vi "everest_loop_test.vi"(1 "error in (no error)":errorcluster, 2 "VISA resource name":refnum<visa-resource-name>="COM3") -> (0 "error out":errorcluster caption="错误输出")   [LabVIEW 2015]
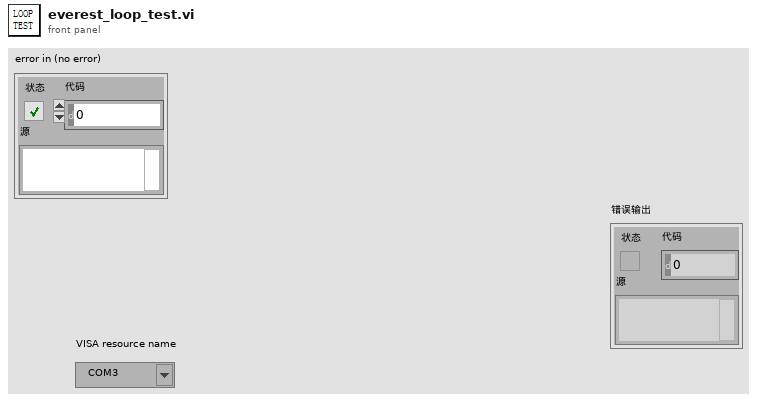
[diagram p1: front panel]
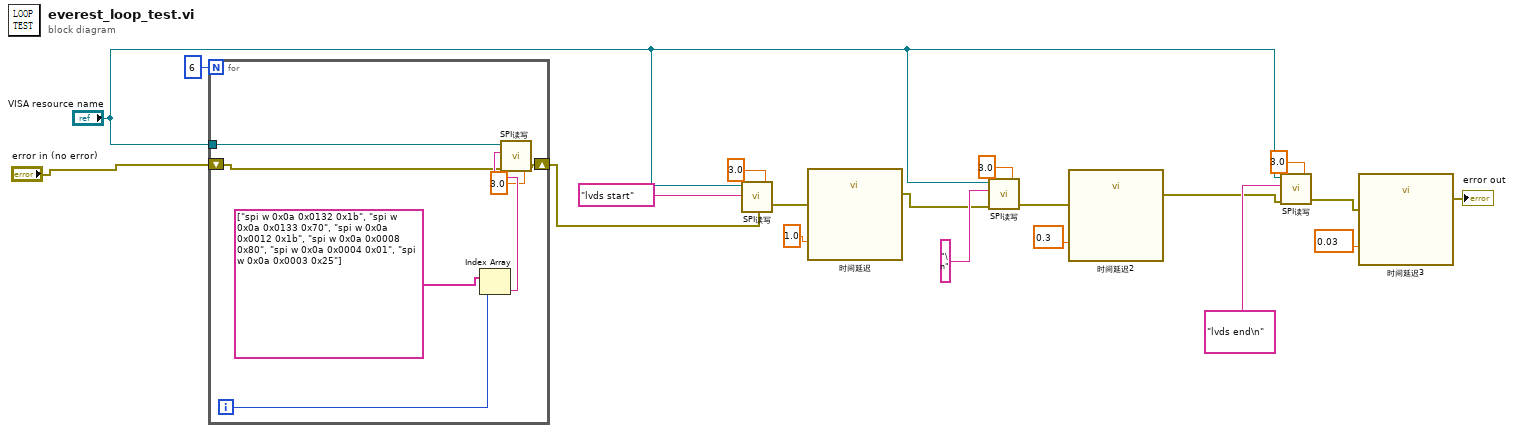
[diagram p0: block diagram]
diagram:
  n1 = for {
    N: 6 -> [_]
    tunnel: "VISA resource name" -> [w23]
    shift-right: [w21] -> w17
    shift-left: "error in (no error)" -> [w22]
    i -> [w25]
    n2 = Index Array(array=string[] ["spi w 0x0a 0x0132 0x1b", "spi w 0x0a 0x0133 0x70", "spi w 0x0a 0x0012 0x1b", "spi w 0x0a 0x0008 0x80", "spi w 0x0a 0x0004 0x01", "spi w 0x0a 0x0003 0x25"], index=w25) -> (element=w24:string)
    n3 = call "SPI读写.vi"("DELAY"=3.0, "error in (no error)"=w22, "往芯片写数据"=w24, "VISA resource name"=w23) -> ("error out"=w21:errorcluster)  [unwired: 1 in, 1 out]
  }
  n4 = call "SPI读写.vi"("DELAY"=3.0, "error in (no error)"=w17, "往芯片写数据"="lvds start", "VISA resource name"="VISA resource name") -> ("error out"=w16:errorcluster)  [unwired: 1 in, 1 out]
  n5 = call "时间延迟"("error in (no error)"=w16, "Delay Time (s)"=1.0) -> ("error out"=w13:errorcluster)  [unwired: 9 in]
  n6 = call "SPI读写.vi"("DELAY"=3.0, "error in (no error)"=w13, "往芯片写数据"="\n", "VISA resource name"="VISA resource name") -> ("error out"=w11:errorcluster)  [unwired: 1 in, 1 out]
  n7 = call "时间延迟2"("error in (no error)"=w11, "Delay Time (s)"=0.3) -> ("error out"=w9:errorcluster)  [unwired: 9 in]
  n8 = call "SPI读写.vi"("DELAY"=3.0, "error in (no error)"=w9, "往芯片写数据"="lvds end\n", "VISA resource name"="VISA resource name") -> ("error out"=w6:errorcluster)  [unwired: 1 in, 1 out]
  n9 = call "时间延迟3"("error in (no error)"=w6, "Delay Time (s)"=0.03) -> ("error out"=→"error out":errorcluster)  [unwired: 9 in]
